vi "DL-Globals.vi"() -> ()   [LabVIEW 2020]
panel:
  in  "Status":enum16{"Idle", "Record", "Error"}(ring)
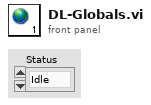
[diagram p1: front panel]
diagram:
